vi "scanner_init.vi"(8 "error in (no error)":errorcluster, 11 "UI in":T1) -> (0 "error out":errorcluster, 3 "UI out":T1)   [LabVIEW 2017]
uses:
  ui.ctl
  ui_buttons.ctl
  types/boc_type.ctl
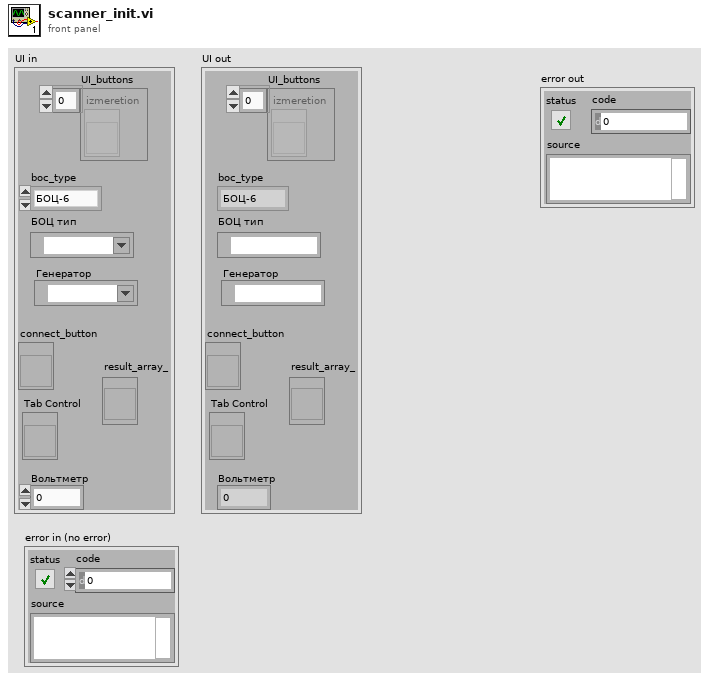
[diagram p1: front panel]
types:
  T1 = typedef "ui.ctl" = cluster{"UI_buttons":T2, "Tab Control":refnum<vi>, "connect_button":refnum<vi>, "generator":refnum<visa-resource-name>, "voltmetr":refnum<visa-resource-name>, "channel_timeout_sec":dbl, "boc_type":T3, "result_array_":refnum<vi>}
  T2 = typedef "ui_buttons.ctl" = refnum<vi>[]
  T3 = typedef "boc_type.ctl" = enum16{"БОЦ-6", "БОЦ-12"}
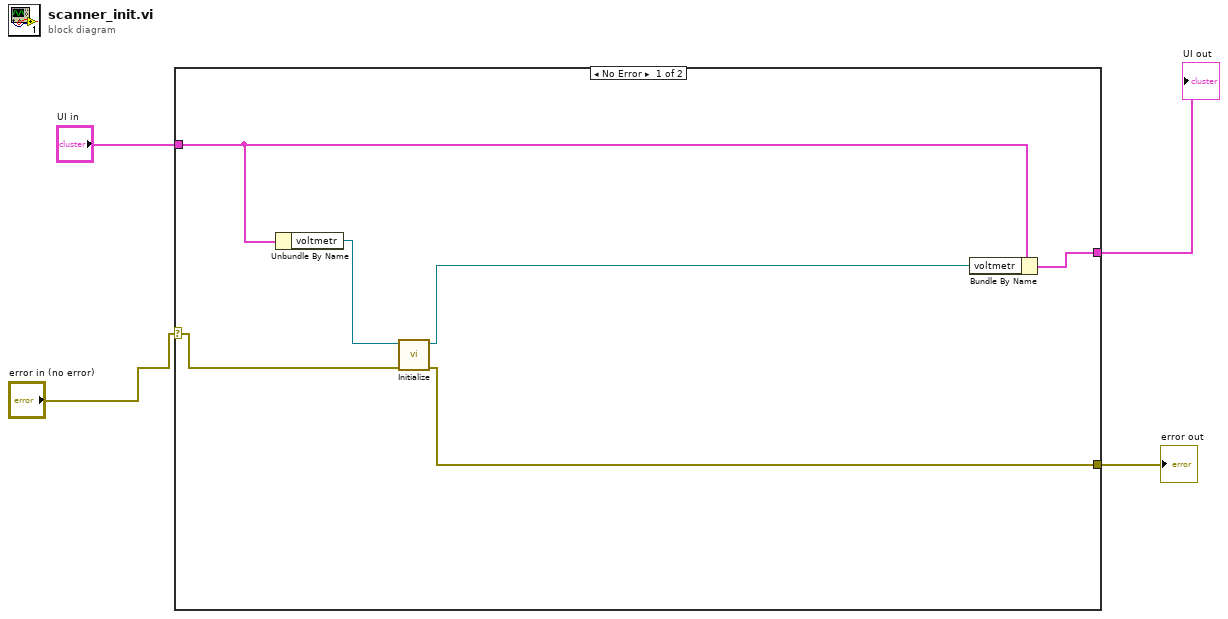
[diagram p0: block diagram]
diagram:
  n1 = case shown="No Error" "error in (no error)" {
    selector: "error in (no error)" -> [w7 w12]
    tunnel: [w10 w11] -> w4
    tunnel: "UI in" -> [w9 w11]
    tunnel: [w5 w12] -> w2
    frame No Error {
      n2 = Unbundle By Name(w9) -> ("voltmetr"=w8:refnum<visa-resource-name>)
      n3 = call <instrlib>:"Initialize.vi"("error in (no error)"=w7, "VISA resource name"=w8) -> ("error out"=w5:errorcluster, "VISA resource name out"=w6:refnum<visa-resource-name>)  [unwired: 7 in, 1 out]
      n4 = Bundle By Name(cluster=w9, "voltmetr"=w6) -> (w10:T1)
    }
    frame Error {
    }
  }
  "UI out" <- w4
  "error out" <- w2
